vi "LightLEDs (SubVI).vi"(9 "Array":bool[](array[boolean]), 10 "LINX Resource":T1) -> ()   [LabVIEW 2014]
uses:
  <vilib>/MakerHub/LINX/Private/Type Defs/LINX Ref.ctl
  <vilib>/MakerHub/LINX/Private/Type Defs/Platform.ctl
  <vilib>/MakerHub/LINX/Private/Type Defs/Interface.ctl
  <vilib>/MakerHub/LINX/Private/Device/Type Defs/LINX Device Config.ctl
  <vilib>/MakerHub/LINX/Private/Device/Type Defs/TCP Config.ctl
  <vilib>/MakerHub/LINX/Private/Device/Type Defs/Channels.ctl
  <vilib>/MakerHub/LINX/Public/Peripherals/Digital/Digital Write 1 Chan.vi
  <vilib>/MakerHub/LINX/Public/Peripherals/Digital/Digital Write N Chans.vi
  <vilib>/MakerHub/LINX/Private/Local IO/LinxDigitalWrite.vi
  <vilib>/MakerHub/LINX/Public/Utilities/Check Channel.vi
  <vilib>/MakerHub/LINX/Private/Local IO/Handle Errors.vi
  <vilib>/MakerHub/LINX/Private/Utilties/Generate Error.vi
  <vilib>/MakerHub/LINX/LMH-LINX.lvlib
  <vilib>/MakerHub/LINX/Private/Device/Device.lvlib
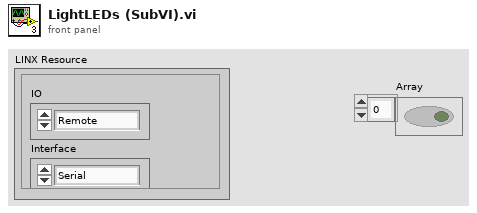
[diagram p1: front panel]
types:
  T1 = typedef "LMH-LINX.lvlib/LINX Ref.ctl" = cluster{"IO":T2, "Interface":T3, "LINX Device Config":T4}
  T2 = typedef "LMH-LINX.lvlib/Platform.ctl" = enum16{"Remote", "Local"}
  T3 = typedef "LMH-LINX.lvlib/Interface.ctl" = enum16{"Serial", "TCP"}
  T4 = typedef "LMH-LINX.lvlib/Device.lvlib/LINX Device Config.ctl" = cluster{"Interface":T3, "COM Port":refnum<visa-resource-name>, "TCP Configuration":T5, "Device Family":u8, "Device ID":u8, "Device Name":string, "TCP Ref":refnum<k5>, "Channels":T6}
  T5 = typedef "LMH-LINX.lvlib/Device.lvlib/TCP Config.ctl" = cluster{"IP Address":string, "Port":u16}
  T6 = typedef "LMH-LINX.lvlib/Channels.ctl" = cluster{"DI":u8[], "DO":u8[], "AI":u8[], "AO":u8[], "PWM":u8[], "QE":u8[], "UART":u8[], "I2C 2":u8[], "SPI":u8[], "CAN":u8[], "Servo":u8[], "AI Ref (V)":dbl, "AI Resolution (Bits)":u8, "AO Ref (V)":dbl, "AO Resolution (Bits)":u8}
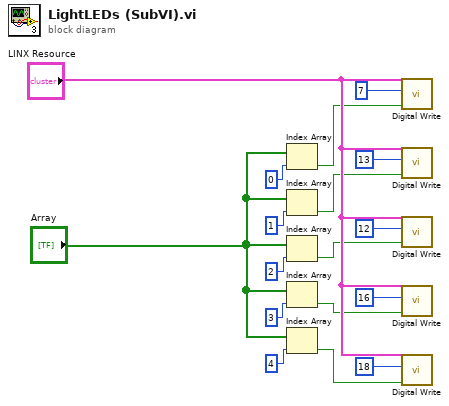
[diagram p0: block diagram]
diagram:
  n1 = Index Array(array="Array", index=0) -> (element=w1:bool)
  n2 = Index Array(array="Array", index=1) -> (element=w2:bool)
  n3 = Index Array(array="Array", index=2) -> (element=w3:bool)
  n4 = Index Array(array="Array", index=3) -> (element=w4:bool)
  n5 = Index Array(array="Array", index=4) -> (element=w5:bool)
  n6 = call-poly <vilib>:"Digital Write.vi"("Output Value"=w1, "DO Channel"=u8 7, "LINX Resource"="LINX Resource") -> ()  [unwired: 7 in, 2 out]
  n7 = call-poly <vilib>:"Digital Write.vi"("Output Value"=w2, "DO Channel"=u8 13, "LINX Resource"="LINX Resource") -> ()  [unwired: 7 in, 2 out]
  n8 = call-poly <vilib>:"Digital Write.vi"("Output Value"=w3, "DO Channel"=u8 12, "LINX Resource"="LINX Resource") -> ()  [unwired: 7 in, 2 out]
  n9 = call-poly <vilib>:"Digital Write.vi"("Output Value"=w4, "DO Channel"=u8 16, "LINX Resource"="LINX Resource") -> ()  [unwired: 7 in, 2 out]
  n10 = call-poly <vilib>:"Digital Write.vi"("Output Value"=w5, "DO Channel"=u8 18, "LINX Resource"="LINX Resource") -> ()  [unwired: 7 in, 2 out]
